vi "DSF.Engine.Plugin.Set Data Type Buffers.vi"(10 "data type buffers":T1, 11 "Plugin in":refnum<class "Plugin.lvclass">) -> (3 "Plugin out":refnum<class "Plugin.lvclass">)   [LabVIEW 2017, in "DSF.Engine.lvlib" / "Plugin.lvclass"]
uses:
  Plugin.lvclass
  Typedefs/DSF.Engine.Typedefs.Type Buffers.ctl
  Plugin.lvclass/Plugin.ctl
  DSF.Engine.lvlib
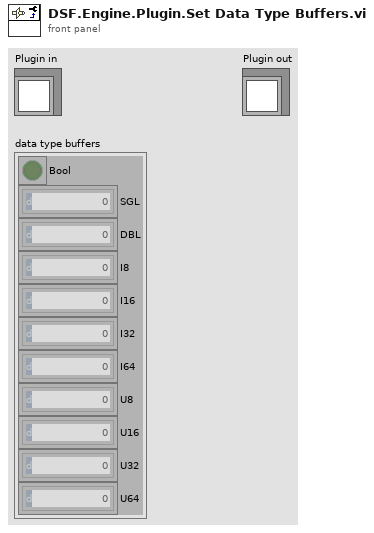
[diagram p1: front panel]
types:
  T1 = typedef "DSF.Engine.lvlib/DSF.Engine.Typedefs.Type Buffers.ctl" = cluster{"Bool":bool[], "SGL":sgl[], "DBL":dbl[], "I8":i8[], "I16":i16[], "I32":i32[], "I64":i64[], "U8":u8[], "U16":u16[], "U32":u32[], "U64":u64[]}
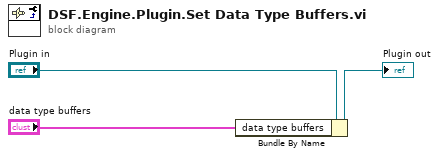
[diagram p0: block diagram]
diagram:
  n1 = Bundle By Name(cluster="Plugin in", "data type buffers"="data type buffers") -> (→"Plugin out":refnum<class "Plugin.lvclass">)
